vi "Importing Model and Setting Light.vi"() -> ()   [LabVIEW 2016]
doc: "This VI demonstrates how to load pre-existent files from VRML and ASE and placing the objects together into a scene."
uses:
  <vilib>/Utility/miscctls.llb/LV3DPointTypeDef.ctl
  <vilib>/picture/3D Picture Control/Object/Create Object (name).vi
  <vilib>/picture/3D Picture Control/Object/Add Object (no reference).vi
  <vilib>/picture/3D Picture Control/Object/Create Object (drawable).vi
  <vilib>/picture/3D Picture Control/Helpers/Set Light (no reference).vi
  <vilib>/picture/3D Picture Control/NI_3D Picture Control.lvlib
panel:
  in  "Light State":enum16{"Inherit Value", "Off", "On"}(ring)=enum."On"
  in  "Stop":bool
  out "3D Picture":refnum<vi>(3d-picture)
  # "Overview: This VI demonstrates how to load VRML (.wrl) and ASE (.ase) files and draw the objects in a 3D Picture.\nRequirements: LabVIEW Full Development System\nInstructions: \n1. Run the VI. This should load two airplanes into the 3D Picture.\n2. You can change the camera view by dragging within the 3D Picture. You can also use SHIFT-drag to zoom in and out of the scene and CTRL-drag to move the scene.\n3. Click Stop to stop the VI."
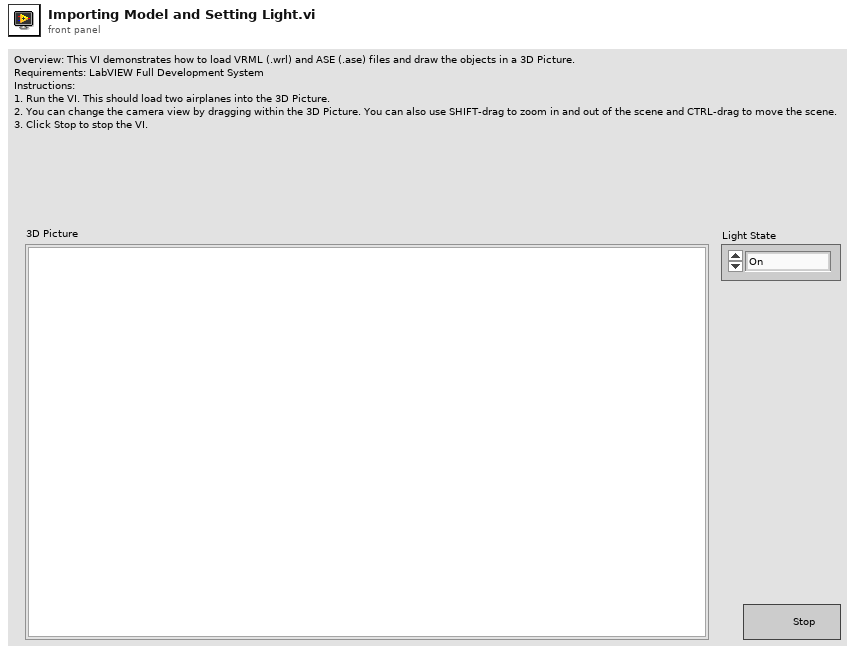
[diagram p1: front panel]
types:
  T1 = typedef "LV3DPointTypeDef.ctl" = cluster{"X":sgl, "Y":sgl, "Z":sgl}
  T2 = enum16{"Inherit Material", "Use entire Material", "Ignore Ambient", "Ignore Diffuse", "Ignore Specular", "Ignore Emission", "Ignore Ambient and Diffuse"}
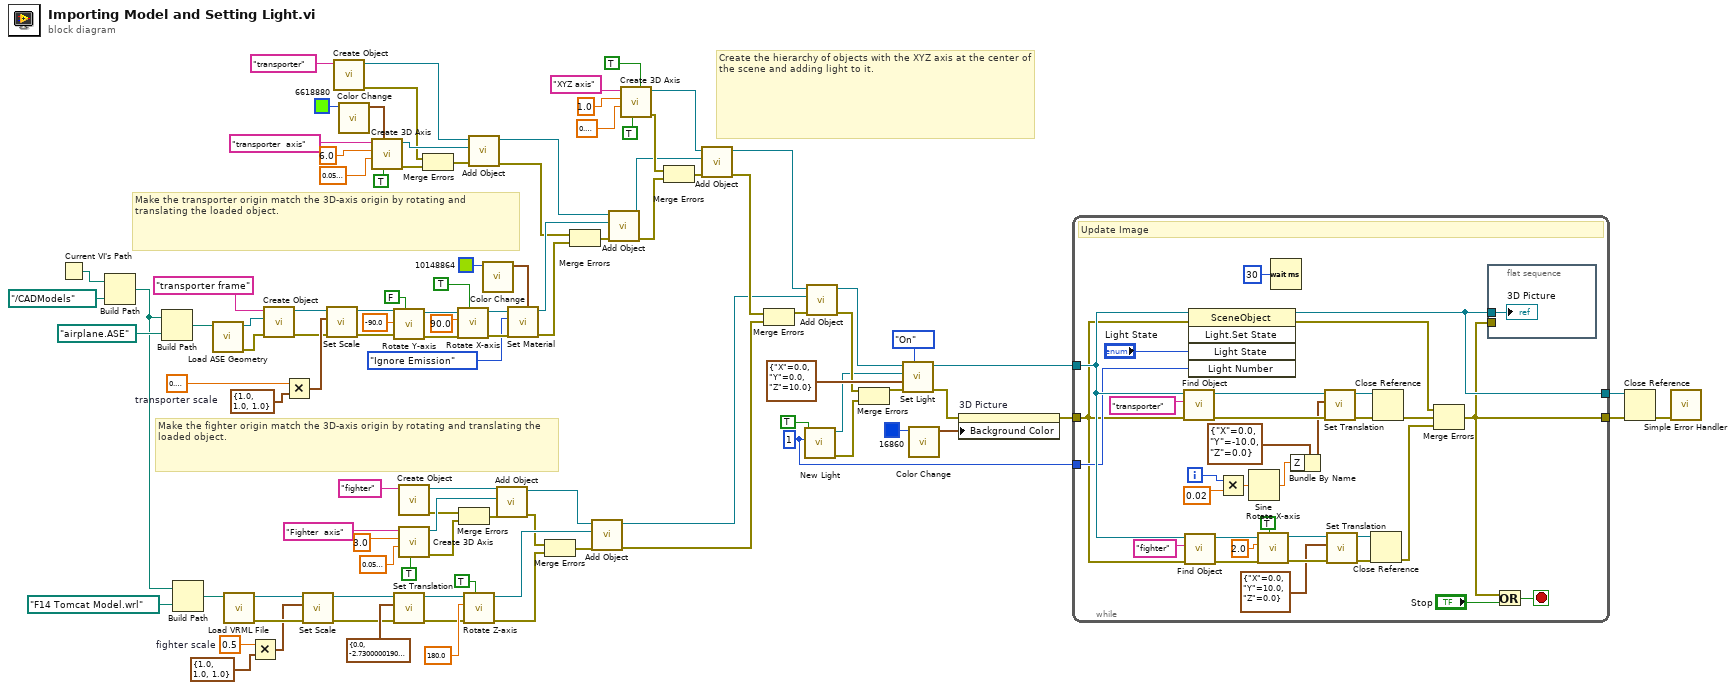
[diagram p0: block diagram]
diagram:
  w84 = sgl 0.5  # fighter scale
  w86 = sgl 0.1  # transporter scale
  w7 = 1 ("Light Number")
  # "Create the hierarchy of objects with the XYZ axis at the center of the scene and adding light to it."
  # "Make the fighter origin match the 3D-axis origin by rotating and translating the loaded object."
  # "Make the transporter origin match the 3D-axis origin by rotating and translating the loaded object."
  n1 = Current VI's Path() -> (path=w5:path)
  n2 = Build Path(base path=w5, name or relative path=path "../CADModels") -> (appended path=w100:path)
  n3 = Build Path(base path=w100, name or relative path=path "airplane.ASE") -> (appended path=w101:path)
  n4 = Build Path(base path=w100, name or relative path=path "F14 Tomcat Model.wrl") -> (appended path=w99:path)
  n5 = call <vilib>:"Load ASE Geometry.vi"("Model File"=w101) -> ("error out"=w25:errorcluster, "New Mesh Refnum"=w104:refnum<vi>)  [unwired: 9 in]
  n6 = call <vilib>:"Load VRML File.vi"("Path"=w99) -> ("error out"=w93:errorcluster, "Scene:Read Scene File"=w92:refnum<vi>)  [unwired: 9 in]
  n7 = Multiply(x=w84, y=cluster{"X":sgl, "Y":sgl, "Z":sgl} {"X"=1.0, "Y"=1.0, "Z"=1.0} ("Scale")) -> (x*y=w85:cluster{"X":sgl, "Y":sgl, "Z":sgl})
  n8 = call-poly <vilib>:"Create Object.vi"("error in (no error)"=w25, "Geometry"=w104, "Name"="transporter frame") -> ("error out"=w45:errorcluster, "Scene:New Object"=w97:refnum<vi>)  [unwired: 7 in]
  n9 = Multiply(x=w86, y=cluster{"X":sgl, "Y":sgl, "Z":sgl} {"X"=1.0, "Y"=1.0, "Z"=1.0} ("Scale")) -> (x*y=w87:cluster{"X":sgl, "Y":sgl, "Z":sgl})
  n10 = call <vilib>:"Set Scale.vi"("error in (no error)"=w93, "Scale"=w85, "Scene Object"=w92) -> ("error out"=w42:errorcluster, "Scaled Object"=w69:refnum<vi>)  [unwired: 7 in]
  n11 = call <vilib>:"Set Scale.vi"("error in (no error)"=w45, "Scale"=w87, "Scene Object"=w97) -> ("error out"=w44:errorcluster, "Scaled Object"=w52:refnum<vi>)  [unwired: 7 in]
  n12 = call-poly <vilib>:"Create Object.vi"("Name"="transporter") -> ("error out"=w10:errorcluster, "Scene:New Object"=w62:refnum<vi>)  [unwired: 9 in]
  n13 = call <vilib>:"Color Change.vi"("Color"=u32 6618880) -> ("RGBA"=w50:cluster{"R":sgl, "G":sgl, "B":sgl, "A":sgl})  [unwired: 10 in]
  n14 = call <vilib>:"Create 3D Axis.vi"("Axis label?"=TRUE, "Color"=w50, "Radius"=sgl 0.05, "Length"=sgl 6.0, "Name"="transporter  axis") -> ("error out"=w11:errorcluster, "New Object Refnum"=w60:refnum<vi>)  [unwired: 5 in]
  n15 = call <vilib>:"Rotate Y-axis.vi"("Relative?"=FALSE, "error in (no error)"=w44, "angle"=-90.0, "Scene Object In"=w52) -> ("error out"=w43:errorcluster, "Scene Object Out"=w48:refnum<vi>)  [unwired: 6 in]
  n16 = call <vilib>:"Set Translation.vi"("error in (no error)"=w42, "Translation"=cluster{"X":sgl, "Y":sgl, "Z":sgl} {"X"=0.0, "Y"=-2.73, "Z"=0.0}, "Scene Object"=w69) -> ("error out"=w41:errorcluster, "Translated Object"=w65:refnum<vi>)  [unwired: 7 in]
  n17 = call-poly <vilib>:"Create Object.vi"("Name"="fighter") -> ("error out"=w14:errorcluster, "Scene:New Object"=w75:refnum<vi>)  [unwired: 9 in]
  n18 = call <vilib>:"Create 3D Axis.vi"("Axis label?"=TRUE, "Radius"=sgl 0.05, "Length"=sgl 3.0, "Name"="Fighter  axis") -> ("error out"=w13:errorcluster, "New Object Refnum"=w78:refnum<vi>)  [unwired: 6 in]
  n19 = Merge Errors(w10, w11) -> (w9:errorcluster)
  n20 = call <vilib>:"Rotate X-axis.vi"("Relative?"=TRUE, "error in (no error)"=w43, "angle"=90.0, "Scene Object In"=w48) -> ("error out"=w40:errorcluster, "Scene Object Out"=w39:refnum<vi>)  [unwired: 6 in]
  n21 = Merge Errors(w14, w13) -> (w12:errorcluster)
  n22 = call <vilib>:"Rotate Z-axis.vi"("Relative?"=TRUE, "error in (no error)"=w41, "angle"=sgl 180.0, "Scene Object In"=w65) -> ("error out"=w36:errorcluster, "Scene Object Out"=w66:refnum<vi>)  [unwired: 6 in]
  n23 = call-poly <vilib>:"Add Object.vi"("error in (no error)"=w9, "New Object In"=w60, "Scene Object In"=w62) -> ("error out"=w31:errorcluster, "Scene Object Out"=w56:refnum<vi>)  [unwired: 7 in]
  n24 = call <vilib>:"Color Change.vi"("Color"=u32 10148864) -> ("RGBA"=w29:cluster{"R":sgl, "G":sgl, "B":sgl, "A":sgl})  [unwired: 10 in]
  n25 = call-poly <vilib>:"Add Object.vi"("error in (no error)"=w12, "New Object In"=w78, "Scene Object In"=w75) -> ("error out"=w35:errorcluster, "Scene Object Out"=w74:refnum<vi>)  [unwired: 7 in]
  n26 = call <vilib>:"Set Material.vi"("Specular"=w29, "error in (no error)"=w40, "Color Mode"=T2."Ignore Emission", "Scene Object In"=w39) -> ("error out"=w32:errorcluster, "Scene Object Out"=w38:refnum<vi>)  [unwired: 6 in]
  n27 = Merge Errors(w35, w36) -> (w34:errorcluster)
  n28 = Merge Errors(w31, w32) -> (w30:errorcluster)
  n29 = call-poly <vilib>:"Add Object.vi"("error in (no error)"=w34, "New Object In"=w66, "Scene Object In"=w74) -> ("error out"=w18:errorcluster, "Scene Object Out"=w19:refnum<vi>)  [unwired: 7 in]
  n30 = call-poly <vilib>:"Add Object.vi"("error in (no error)"=w30, "New Object In"=w38, "Scene Object In"=w56) -> ("error out"=w17:errorcluster, "Scene Object Out"=w16:refnum<vi>)  [unwired: 7 in]
  n31 = call <vilib>:"Create 3D Axis.vi"("Half plane?"=TRUE, "Axis label?"=TRUE, "Radius"=sgl 0.1, "Length"=sgl 1.0, "Name"="XYZ axis") -> ("error out"=w24:errorcluster, "New Object Refnum"=w55:refnum<vi>)  [unwired: 5 in]
  n32 = Merge Errors(w24, w17) -> (w23:errorcluster)
  n33 = call-poly <vilib>:"Add Object.vi"("error in (no error)"=w23, "New Object In"=w16, "Scene Object In"=w55) -> ("error out"=w27:errorcluster, "Scene Object Out"=w54:refnum<vi>)  [unwired: 7 in]
  n34 = Merge Errors(w27, w18) -> (w26:errorcluster)
  n35 = call <vilib>:"New Light.vi"("Light Number"=w7, "At Infinity"=TRUE) -> ("error out"=w22:errorcluster, "New Light Refnum"=w8:refnum<vi>)  [unwired: 8 in]
  n36 = call-poly <vilib>:"Add Object.vi"("error in (no error)"=w26, "New Object In"=w19, "Scene Object In"=w54) -> ("error out"=w21:errorcluster, "Scene Object Out"=w77:refnum<vi>)  [unwired: 7 in]
  n37 = Merge Errors(w21, w22) -> (w20:errorcluster)
  n38 = call-poly <vilib>:"Set Light.vi"("Light State"=enum16{"Inherit Value", "Off", "On"}."On", "error in (no error)"=w20, "Position"=T1 {"X"=0.0, "Y"=0.0, "Z"=10.0}, "Light Refnum In"=w8, "Scene Object In"=w77) -> ("error out"=w15:errorcluster, "Scene Object Out"=w4:refnum<vi>)  [unwired: 5 in]
  n39 = call <vilib>:"Color Change.vi"("Color"=u32 16860) -> ("RGBA"=w91:cluster{"R":sgl, "G":sgl, "B":sgl, "A":sgl})  [unwired: 10 in]
  n40 = property on="3D Picture" class="SceneGraphDisp (strict)"(error in=w15, "Background Color"=w91) -> (error out=w6:errorcluster)  [unwired: 1 in, 1 out]
  n41 = while {
    tunnel: w4 -> [w117]
    tunnel: w6 -> [w113]
    tunnel: [w105] -> w3
    tunnel: w7 -> [w116]
    tunnel: [w106] -> w1
    i -> [w122]
    stop <- w124 stop-if-true
    # "Update Image"
    n42 = call <vilib>:"Find Object.vi"("error in (no error)"=w113, "Object Name"="transporter", "Scene Refnum"=w117) -> ("error out"=w132:errorcluster, "Object Refnum"=w131:refnum<vi>)  [unwired: 7 in]
    n43 = call <vilib>:"Find Object.vi"("error in (no error)"=w113, "Object Name"="fighter", "Scene Refnum"=w117) -> ("error out"=w127:errorcluster, "Object Refnum"=w128:refnum<vi>)  [unwired: 7 in]
    n44 = invoke class="SceneObject" method="Light.Set State"(reference=w117, error in=w113, "Light State"="Light State", "Light Number"=w116) -> (reference out=w106:refnum<vi>, error out=w114:errorcluster)  [unwired: 1 in, 3 out]
    n45 = Multiply(x=w122, y=0.02) -> (x*y=w119:dbl)
    n46 = Sine(x=w119) -> (sin(x)=w120:dbl)
    n47 = call <vilib>:"Rotate X-axis.vi"("Relative?"=TRUE, "error in (no error)"=w127, "angle"=2.0, "Scene Object In"=w128) -> ("error out"=w129:errorcluster, "Scene Object Out"=w130:refnum<vi>)  [unwired: 6 in]
    n48 = Wait (ms)(milliseconds to wait=u32 30) -> ()  [unwired: 1 out]
    n49 = Bundle By Name(cluster=cluster{"X":sgl, "Y":sgl, "Z":sgl} {"X"=0.0, "Y"=-10.0, "Z"=0.0} ("Translation"), "Z"=w120) -> (w121:cluster{"X":sgl, "Y":sgl, "Z":sgl})
    n50 = call <vilib>:"Set Translation.vi"("error in (no error)"=w132, "Translation"=w121, "Scene Object"=w131) -> ("error out"=w111:errorcluster, "Translated Object"=w110:refnum<vi>)  [unwired: 7 in]
    n51 = call <vilib>:"Set Translation.vi"("error in (no error)"=w129, "Translation"=cluster{"X":sgl, "Y":sgl, "Z":sgl} {"X"=0.0, "Y"=10.0, "Z"=0.0}, "Scene Object"=w130) -> ("error out"=w125:errorcluster, "Translated Object"=w107:refnum<vi>)  [unwired: 7 in]
    n52 = Close Reference(reference=w107, error in (no error)=w125) -> (error out=w108:errorcluster)
    n53 = Close Reference(reference=w110, error in (no error)=w111) -> (error out=w109:errorcluster)
    n54 = Merge Errors(w114, w109, w108) -> (w105:errorcluster)
    n55 = flat-sequence {
      tunnel: w106 -> [w138]
      tunnel: w105 -> [_]
      frame #0 {
        "3D Picture" <- w138
      }
    }
    n56 = Or(x=w105, y="Stop") -> (x .or. y?=w124:bool)
  }
  n57 = Close Reference(reference=w1, error in (no error)=w3) -> (error out=w2:errorcluster)
  n58 = call <vilib>:"Simple Error Handler.vi"("error in (no error)"=w2) -> ()  [unwired: 4 in, 5 out]
